vi "QCA Global.vi"() -> ()   [LabVIEW 2019]
panel:
  in  "Channel File":path=path "G:/b28/NMR program/B28_Normal_NMR.txt"
  in  "Monitor Delay":i32
  in  "Data Suppliers":string[](array[string])
  in  "QMeterTempChan":i32=1
  in  "DCLevelChan":i32=1
  in  "Dry Run":bool
  in  "ScanGain":i32=1
  in  "ScanDACChan":i32
  in  "Channel Type Info":T1(array[cluster])=[{"Name"="ScanSweeps", "Type"=enum."I32", "Changeable"=TRUE}, {"Name"="ScanSteps", "Type"=enum."I32", "Changeable"=FALSE}, {"Name"="ScanFreq", "Type"=enum."I32", "Changeable"=FALSE}, {"Name"="ScanIntv", "Type"=enum."I32", "Changeable"=FALSE}, {"Name"="RFFreq", "Type"=enum."DBL", "Changeable"=TRUE}, {"Name"="RFMod", "Type"=enum."I32", "Changeable"=TRUE}, {"Name"="RFPower", "Type"=enum."I32", "Changeable"=TRUE}, {"Name"="YaleGain", "Type"=enum."I32", "Changeable"=TRUE}, {"Name"="QMeterNum", "Type"=enum."I32", "Changeable"=FALSE}, {"Name"="QMeterName", "Type"=enum."STR", "Changeable"=FALSE}, {"Name"="CalConst", "Type"=enum."DBL", "Changeable"=TRUE}, {"Name"="Baseline", "Type"=enum."I32", "Changeable"=TRUE}, {"Name"="ScanGain", "Type"=enum."I32", "Changeable"=TRUE}, {"Name"="ScanADCChan", "Type"=enum."I32", "Changeable"=FALSE}, {"Name"="ScanDACChan", "Type"=enum."I32", "Changeable"=FALSE}, {"Name"="Material", "Type"=enum."STR", "Changeable"=FALSE}, {"Name"="DCLevelChan", "Type"=enum."I32", "Changeable"=FALSE}, {"Name"="QMeterTempChan", "Type"=enum."I32", "Changeable"=FALSE}]
  in  "Channel Array":string[][][](array[string])=[[["ChanName", "Top Deuteron"], ["ScanSweeps", "200"], ["ScanSteps", "500"], ["ScanFreq", "15287"], ["ScanIntv", "100"], ["RFFreq", "3.270000E+1"], ["RFMod", "400"], ["RFPower", "280"], ["YaleGain", "1"], ["QMeterNum", "2"], ["QMeterName", "Top Deuteron"], ["CalConst", "-6.550000E+0"], ["Baseline", "1000761086"], ["ScanGain", "1"], ["ScanADCChan", "1"], ["ScanDACChan", "0"], ["Material", "15ND3"]], [["ChanName", "Bottom Deuteron"], ["ScanSweeps", "200"], ["ScanSteps", "500"], ["ScanFreq", "15287"], ["ScanIntv", "100"], ["RFFreq", "3.270000E+1"], ["RFMod", "400"], ["RFPower", "280"], ["YaleGain", "1"], ["QMeterNum", "4"], ["QMeterName", "Bottom Deuteron"], ["CalConst", "-6.762000E+0"], ["Baseline", "1000746959"], ["ScanGain", "1"], ["ScanADCChan", "3"], ["ScanDACChan", "0"], ["Material", "15ND3"]], [["ChanName", "Top Proton"], ["ScanSweeps", "100"], ["ScanSteps", "500"], ["ScanFreq", "10000"], ["ScanIntv", "100"], ["RFFreq", "2.130000E+2"], ["RFMod", "400"], ["RFPower", "280"], ["YaleGain", "0"], ["QMeterNum", "1"], ["QMeterName", "Top Proton"], ["CalConst", "6.441300E-1"], ["Baseline", "996305333"], ["ScanGain", "1"], ["ScanADCChan", "0"], ["ScanDACChan", "0"], ["Material", "15NH3"]], [["ChanName", "Bottom Proton"], ["ScanSweeps", "100"], ["ScanSteps", "500"], ["ScanFreq", "10000"], ["ScanIntv", "100"], ["RFFreq", "2.130000E+2"], ["RFMod", "400"], ["RFPower", "280"], ["YaleGain", "0"], ["QMeterNum", "3"], ["QMeterName", "Bottom Proton"], ["CalConst", "3.000000E+0"], ["Baseline", "987786192"], ["ScanGain", "1"], ["ScanADCChan", "2"], ["ScanDACChan", "0"], ["Material", "15NH3"]]]
  in  "Fake Signal Height":dbl format="%.2f"
  in  "Baseline":i32=1000761086
  in  "CalConst":dbl=-6.55 format="%.3e"
  in  "ScanADCChan":i32=1
  in  "ScanRamp":dbl[](array[numeric])=[-1.0, -0.996, -0.992, -0.988, -0.984, -0.98, -0.976, -0.972, -0.968, -0.964, -0.96, -0.956, -0.952, -0.948, -0.944, -0.94, -0.9359999999999999, -0.9319999999999999, -0.928, -0.924, -0.92, -0.916, -0.912, -0.908, -0.904, -0.9, -0.896, -0.892, -0.888, -0.884, -0.88, -0.876, -0.872, -0.868, -0.864, -0.86, -0.856, -0.852, -0.848, -0.844, -0.84, -0.836, -0.832, -0.8280000000000001, -0.8240000000000001, -0.8200000000000001, -0.8160000000000001, -0.812, -0.808, -0.804, -0.8, -0.796, -0.792, -0.788, -0.784, -0.78, -0.776, -0.772, -0.768, -0.764, -0.76, -0.756, -0.752, -0.748, -0.744, -0.74, -0.736, -0.732, -0.728, -0.724, -0.72, -0.716, -0.712, -0.708, -0.704, -0.7, -0.696, -0.692, -0.688, -0.6839999999999999, -0.6799999999999999, -0.6759999999999999, -0.6719999999999999, -0.6679999999999999, -0.6639999999999999, -0.6599999999999999, -0.656, -0.652, -0.648, -0.644, -0.64, -0.636, -0.632, -0.628, -0.624, -0.62, -0.616, -0.612, -0.608, -0.604, -0.6, -0.596, -0.5920000000000001, -0.5880000000000001, -0.5840000000000001, -0.5800000000000001, -0.5760000000000001, -0.5720000000000001, -0.5680000000000001, -0.5640000000000001, -0.56, -0.556, -0.552, -0.548, -0.544, -0.54, -0.536, -0.532, -0.528, -0.524, -0.52, -0.516, -0.512, -0.508, -0.504, -0.5, -0.496, -0.492, -0.488, -0.484, -0.48, -0.476, -0.472, -0.46799999999999997, -0.46399999999999997, -0.45999999999999996, -0.45599999999999996, -0.45199999999999996, -0.44799999999999995, -0.44399999999999995, -0.43999999999999995, -0.43600000000000005, -0.43200000000000005, -0.42800000000000005, -0.42400000000000004, -0.42000000000000004, -0.41600000000000004, -0.41200000000000003, -0.40800000000000003, -0.404, -0.4, -0.396, -0.392, -0.388, -0.384, -0.38, -0.376, -0.372, -0.368, -0.364, -0.36, -0.356, -0.352, -0.348, -0.344, -0.33999999999999997, -0.33599999999999997, -0.33199999999999996, -0.32799999999999996, -0.32399999999999995, -0.31999999999999995, -0.31599999999999995, -0.31200000000000006, -0.30800000000000005, -0.30400000000000005, -0.30000000000000004, -0.29600000000000004, -0.29200000000000004, -0.28800000000000003, -0.28400000000000003, -0.28, -0.276, -0.272, -0.268, -0.264, -0.26, -0.256, -0.252, -0.248, -0.244, -0.24, -0.236, -0.23199999999999998, -0.22799999999999998, -0.22399999999999998, -0.21999999999999997, -0.21599999999999997, -0.21199999999999997, -0.20799999999999996, -0.20399999999999996, -0.19999999999999996, -0.19599999999999995, -0.19199999999999995, -0.18799999999999994, -0.18400000000000005, -0.18000000000000005, -0.17600000000000005, -0.17200000000000004, -0.16800000000000004, -0.16400000000000003, -0.16000000000000003, -0.15600000000000003, -0.15200000000000002, -0.14800000000000002, -0.14400000000000002, -0.14, -0.136, -0.132, -0.128, -0.124, -0.12, -0.11599999999999999, -0.11199999999999999, -0.10799999999999998, -0.10399999999999998, -0.09999999999999998, -0.09599999999999997, -0.09199999999999997, -0.08799999999999997, -0.08399999999999996, -0.07999999999999996, -0.07599999999999996, -0.07199999999999995, -0.06799999999999995, -0.06399999999999995, -0.06000000000000005, -0.05600000000000005, -0.052000000000000046, -0.04800000000000004, -0.04400000000000004, -0.040000000000000036, -0.03600000000000003, -0.03200000000000003, -0.028000000000000025, -0.02400000000000002, -0.020000000000000018, -0.016000000000000014, -0.01200000000000001, -0.008000000000000007, -0.0040000000000000036, 0.0, 0.0040000000000000036, 0.008000000000000007, 0.01200000000000001, 0.016000000000000014, 0.020000000000000018, 0.02400000000000002, 0.028000000000000025, 0.03200000000000003, 0.03600000000000003, 0.040000000000000036, 0.04400000000000004, 0.04800000000000004, 0.052000000000000046, 0.05600000000000005, 0.06000000000000005, 0.06400000000000006, 0.06800000000000006, 0.07200000000000006, 0.07600000000000007, 0.08000000000000007, 0.08400000000000007, 0.08800000000000008, 0.09200000000000008, 0.09600000000000009, 0.10000000000000009, 0.10400000000000009, 0.1080000000000001, 0.1120000000000001, 0.1160000000000001, 0.1200000000000001, 0.12400000000000011, 0.1279999999999999, 0.1319999999999999, 0.1359999999999999, 0.1399999999999999, 0.1439999999999999, 0.1479999999999999, 0.1519999999999999, 0.15599999999999992, 0.15999999999999992, 0.16399999999999992, 0.16799999999999993, 0.17199999999999993, 0.17599999999999993, 0.17999999999999994, 0.18399999999999994, 0.18799999999999994, 0.19199999999999995, 0.19599999999999995, 0.19999999999999996, 0.20399999999999996, 0.20799999999999996, 0.21199999999999997, 0.21599999999999997, 0.21999999999999997, 0.22399999999999998, 0.22799999999999998, 0.23199999999999998, 0.236, 0.24, 0.244, 0.248, 0.252, 0.256, 0.26, 0.264, 0.268, 0.272, 0.276, 0.28, 0.28400000000000003, 0.28800000000000003, 0.29200000000000004, 0.29600000000000004, 0.30000000000000004, 0.30400000000000005, 0.30800000000000005, 0.31200000000000006, 0.31600000000000006, 0.32000000000000006, 0.32400000000000007, 0.32800000000000007, 0.3320000000000001, 0.3360000000000001, 0.3400000000000001, 0.3440000000000001, 0.3480000000000001, 0.3520000000000001, 0.3560000000000001, 0.3600000000000001, 0.3640000000000001, 0.3680000000000001, 0.3720000000000001, 0.3759999999999999, 0.3799999999999999, 0.3839999999999999, 0.3879999999999999, 0.3919999999999999, 0.3959999999999999, 0.3999999999999999, 0.4039999999999999, 0.4079999999999999, 0.4119999999999999, 0.4159999999999999, 0.41999999999999993, 0.42399999999999993, 0.42799999999999994, 0.43199999999999994, 0.43599999999999994, 0.43999999999999995, 0.44399999999999995, 0.44799999999999995, 0.45199999999999996, 0.45599999999999996, 0.45999999999999996, 0.46399999999999997, 0.46799999999999997, 0.472, 0.476, 0.48, 0.484, 0.488, 0.492, 0.496, 0.5, 0.504, 0.508, 0.512, 0.516, 0.52, 0.524, 0.528, 0.532, 0.536, 0.54, 0.544, 0.548, 0.552, 0.556, 0.56, 0.5640000000000001, 0.5680000000000001, 0.5720000000000001, 0.5760000000000001, 0.5800000000000001, 0.5840000000000001, 0.5880000000000001, 0.5920000000000001, 0.5960000000000001, 0.6000000000000001, 0.6040000000000001, 0.6080000000000001, 0.6120000000000001, 0.6160000000000001, 0.6200000000000001, 0.6240000000000001, 0.6279999999999999, 0.6319999999999999, 0.6359999999999999, 0.6399999999999999, 0.6439999999999999, 0.6479999999999999, 0.6519999999999999, 0.6559999999999999, 0.6599999999999999, 0.6639999999999999, 0.6679999999999999, 0.6719999999999999, 0.6759999999999999, 0.6799999999999999, 0.6839999999999999, 0.688, 0.692, 0.696, 0.7, 0.704, 0.708, 0.712, 0.716, 0.72, 0.724, 0.728, 0.732, 0.736, 0.74, 0.744, 0.748, 0.752, 0.756, 0.76, 0.764, 0.768, 0.772, 0.776, 0.78, 0.784, 0.788, 0.792, 0.796, 0.8, 0.804, 0.808, 0.812, 0.8160000000000001, 0.8200000000000001, 0.8240000000000001, 0.8280000000000001, 0.8320000000000001, 0.8360000000000001, 0.8400000000000001, 0.8440000000000001, 0.8480000000000001, 0.8520000000000001, 0.8560000000000001, 0.8600000000000001, 0.8640000000000001, 0.8680000000000001, 0.8720000000000001, 0.8759999999999999, 0.8799999999999999, 0.8839999999999999, 0.8879999999999999, 0.8919999999999999, 0.8959999999999999, 0.8999999999999999, 0.9039999999999999, 0.9079999999999999, 0.9119999999999999, 0.9159999999999999, 0.9199999999999999, 0.9239999999999999, 0.9279999999999999, 0.9319999999999999, 0.9359999999999999, 0.94, 0.944, 0.948, 0.952, 0.956, 0.96, 0.964, 0.968, 0.972, 0.976, 0.98, 0.984, 0.988, 0.992, 0.996, 0.996, 0.992, 0.988, 0.984, 0.98, 0.976, 0.972, 0.968, 0.964, 0.96, 0.956, 0.952, 0.948, 0.944, 0.94, 0.9359999999999999, 0.9319999999999999, 0.9279999999999999, 0.9239999999999999, 0.9199999999999999, 0.9159999999999999, 0.9119999999999999, 0.9079999999999999, 0.9039999999999999, 0.8999999999999999, 0.8959999999999999, 0.8919999999999999, 0.8879999999999999, 0.8839999999999999, 0.8799999999999999, 0.8759999999999999, 0.8720000000000001, 0.8680000000000001, 0.8640000000000001, 0.8600000000000001, 0.8560000000000001, 0.8520000000000001, 0.8480000000000001, 0.8440000000000001, 0.8400000000000001, 0.8360000000000001, 0.8320000000000001, 0.8280000000000001, 0.8240000000000001, 0.8200000000000001, 0.8160000000000001, 0.812, 0.808, 0.804, 0.8, 0.796, 0.792, 0.788, 0.784, 0.78, 0.776, 0.772, 0.768, 0.764, 0.76, 0.756, 0.752, 0.748, 0.744, 0.74, 0.736, 0.732, 0.728, 0.724, 0.72, 0.716, 0.712, 0.708, 0.704, 0.7, 0.696, 0.692, 0.688, 0.6839999999999999, 0.6799999999999999, 0.6759999999999999, 0.6719999999999999, 0.6679999999999999, 0.6639999999999999, 0.6599999999999999, 0.6559999999999999, 0.6519999999999999, 0.6479999999999999, 0.6439999999999999, 0.6399999999999999, 0.6359999999999999, 0.6319999999999999, 0.6279999999999999, 0.6240000000000001, 0.6200000000000001, 0.6160000000000001, 0.6120000000000001, 0.6080000000000001, 0.6040000000000001, 0.6000000000000001, 0.5960000000000001, 0.5920000000000001, 0.5880000000000001, 0.5840000000000001, 0.5800000000000001, 0.5760000000000001, 0.5720000000000001, 0.5680000000000001, 0.5640000000000001, 0.56, 0.556, 0.552, 0.548, 0.544, 0.54, 0.536, 0.532, 0.528, 0.524, 0.52, 0.516, 0.512, 0.508, 0.504, 0.5, 0.496, 0.492, 0.488, 0.484, 0.48, 0.476, 0.472, 0.46799999999999997, 0.46399999999999997, 0.45999999999999996, 0.45599999999999996, 0.45199999999999996, 0.44799999999999995, 0.44399999999999995, 0.43999999999999995, 0.43599999999999994, 0.43199999999999994, 0.42799999999999994, 0.42399999999999993, 0.41999999999999993, 0.4159999999999999, 0.4119999999999999, 0.4079999999999999, 0.4039999999999999, 0.3999999999999999, 0.3959999999999999, 0.3919999999999999, 0.3879999999999999, 0.3839999999999999, 0.3799999999999999, 0.3759999999999999, 0.3720000000000001, 0.3680000000000001, 0.3640000000000001, 0.3600000000000001, 0.3560000000000001, 0.3520000000000001, 0.3480000000000001, 0.3440000000000001, 0.3400000000000001, 0.3360000000000001, 0.3320000000000001, 0.32800000000000007, 0.32400000000000007, 0.32000000000000006, 0.31600000000000006, 0.31200000000000006, 0.30800000000000005, 0.30400000000000005, 0.30000000000000004, 0.29600000000000004, 0.29200000000000004, 0.28800000000000003, 0.28400000000000003, 0.28, 0.276, 0.272, 0.268, 0.264, 0.26, 0.256, 0.252, 0.248, 0.244, 0.24, 0.236, 0.23199999999999998, 0.22799999999999998, 0.22399999999999998, 0.21999999999999997, 0.21599999999999997, 0.21199999999999997, 0.20799999999999996, 0.20399999999999996, 0.19999999999999996, 0.19599999999999995, 0.19199999999999995, 0.18799999999999994, 0.18399999999999994, 0.17999999999999994, 0.17599999999999993, 0.17199999999999993, 0.16799999999999993, 0.16399999999999992, 0.15999999999999992, 0.15599999999999992, 0.1519999999999999, 0.1479999999999999, 0.1439999999999999, 0.1399999999999999, 0.1359999999999999, 0.1319999999999999, 0.1279999999999999, 0.12400000000000011, 0.1200000000000001, 0.1160000000000001, 0.1120000000000001, 0.1080000000000001, 0.10400000000000009, 0.10000000000000009, 0.09600000000000009, 0.09200000000000008, 0.08800000000000008, 0.08400000000000007, 0.08000000000000007, 0.07600000000000007, 0.07200000000000006, 0.06800000000000006, 0.06400000000000006, 0.06000000000000005, 0.05600000000000005, 0.052000000000000046, 0.04800000000000004, 0.04400000000000004, 0.040000000000000036, 0.03600000000000003, 0.03200000000000003, 0.028000000000000025, 0.02400000000000002, 0.020000000000000018, 0.016000000000000014, 0.01200000000000001, 0.008000000000000007, 0.0040000000000000036, 0.0, -0.0040000000000000036, -0.008000000000000007, -0.01200000000000001, -0.016000000000000014, -0.020000000000000018, -0.02400000000000002, -0.028000000000000025, -0.03200000000000003, -0.03600000000000003, -0.040000000000000036, -0.04400000000000004, -0.04800000000000004, -0.052000000000000046, -0.05600000000000005, -0.06000000000000005, -0.06399999999999995, -0.06799999999999995, -0.07199999999999995, -0.07599999999999996, -0.07999999999999996, -0.08399999999999996, -0.08799999999999997, -0.09199999999999997, -0.09599999999999997, -0.09999999999999998, -0.10399999999999998, -0.10799999999999998, -0.11199999999999999, -0.11599999999999999, -0.12, -0.124, -0.128, -0.132, -0.136, -0.14, -0.14400000000000002, -0.14800000000000002, -0.15200000000000002, -0.15600000000000003, -0.16000000000000003, -0.16400000000000003, -0.16800000000000004, -0.17200000000000004, -0.17600000000000005, -0.18000000000000005, -0.18400000000000005, -0.18799999999999994, -0.19199999999999995, -0.19599999999999995, -0.19999999999999996, -0.20399999999999996, -0.20799999999999996, -0.21199999999999997, -0.21599999999999997, -0.21999999999999997, -0.22399999999999998, -0.22799999999999998, -0.23199999999999998, -0.236, -0.24, -0.244, -0.248, -0.252, -0.256, -0.26, -0.264, -0.268, -0.272, -0.276, -0.28, -0.28400000000000003, -0.28800000000000003, -0.29200000000000004, -0.29600000000000004, -0.30000000000000004, -0.30400000000000005, -0.30800000000000005, -0.31200000000000006, -0.31599999999999995, -0.31999999999999995, -0.32399999999999995, -0.32799999999999996, -0.33199999999999996, -0.33599999999999997, -0.33999999999999997, -0.344, -0.348, -0.352, -0.356, -0.36, -0.364, -0.368, -0.372, -0.376, -0.38, -0.384, -0.388, -0.392, -0.396, -0.4, -0.404, -0.40800000000000003, -0.41200000000000003, -0.41600000000000004, -0.42000000000000004, -0.42400000000000004, -0.42800000000000005, -0.43200000000000005, -0.43600000000000005, -0.43999999999999995, -0.44399999999999995, -0.44799999999999995, -0.45199999999999996, -0.45599999999999996, -0.45999999999999996, -0.46399999999999997, -0.46799999999999997, -0.472, -0.476, -0.48, -0.484, -0.488, -0.492, -0.496, -0.5, -0.504, -0.508, -0.512, -0.516, -0.52, -0.524, -0.528, -0.532, -0.536, -0.54, -0.544, -0.548, -0.552, -0.556, -0.56, -0.5640000000000001, -0.5680000000000001, -0.5720000000000001, -0.5760000000000001, -0.5800000000000001, -0.5840000000000001, -0.5880000000000001, -0.5920000000000001, -0.596, -0.6, -0.604, -0.608, -0.612, -0.616, -0.62, -0.624, -0.628, -0.632, -0.636, -0.64, -0.644, -0.648, -0.652, -0.656, -0.6599999999999999, -0.6639999999999999, -0.6679999999999999, -0.6719999999999999, -0.6759999999999999, -0.6799999999999999, -0.6839999999999999, -0.688, -0.692, -0.696, -0.7, -0.704, -0.708, -0.712, -0.716, -0.72, -0.724, -0.728, -0.732, -0.736, -0.74, -0.744, -0.748, -0.752, -0.756, -0.76, -0.764, -0.768, -0.772, -0.776, -0.78, -0.784, -0.788, -0.792, -0.796, -0.8, -0.804, -0.808, -0.812, -0.8160000000000001, -0.8200000000000001, -0.8240000000000001, -0.8280000000000001, -0.832, -0.836, -0.84, -0.844, -0.848, -0.852, -0.856, -0.86, -0.864, -0.868, -0.872, -0.876, -0.88, -0.884, -0.888, -0.892, -0.896, -0.9, -0.904, -0.908, -0.912, -0.916, -0.92, -0.924, -0.928, -0.9319999999999999, -0.9359999999999999, -0.94, -0.944, -0.948, -0.952, -0.956, -0.96, -0.964, -0.968, -0.972, -0.976, -0.98, -0.984, -0.988, -0.992, -0.996, -1.0] format="%.2f"
  in  "ScanDevice":i32=1
  in  "QMeterNum":i32=2
  in  "QMeterChans":string="2,3,4,5,6,7"
  in  "QMeterDevice":i32=2
  in  "YaleChans":string="8,9,10"
  in  "YaleDevice":i16=2
  in  "RFDevice":i32=28
  in  "QMeterName":string="Top Deuteron"
  in  "YaleGain":i32=1
  in  "RFPower":i32=280
  in  "RFMod":i32=400
  in  "RFFreq":dbl=32.7 format="%.3f"
  in  "ScanFreq":i32=15287
  in  "ScanSteps":i32=500
  in  "ChanName":string="Top Deuteron"
  in  "ScanSweeps":i32=200
  in  "Current Channel":i32
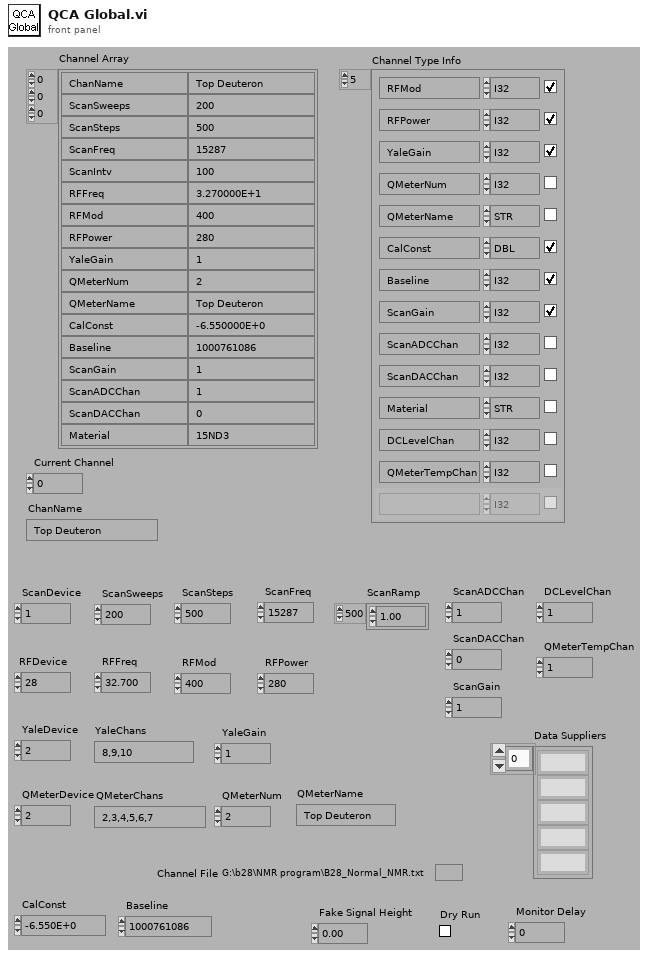
[diagram p1: front panel]
types:
  T1 = cluster{"Name":string, "Type":enum16{"I32", "DBL", "STR"}, "Changeable":bool}[]
diagram:
